vi "Line IR Read.vi"() -> (0 "Line IR Right":bool, 1 "Line IR Left":bool)   [LabVIEW 2013]
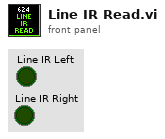
[diagram p1: front panel]
types:
  T1 = typedef "WPI_DigitalInputDevRef.ctl" = cluster{"DevStatus":errorcluster, "DIO Channel":T2, "Digital Module":T3}
  T2 = typedef "FPGA_DIOChannel.ctl" = enum8{"DIO 1", "DIO 2", "DIO 3", "DIO 4", "DIO 5", "DIO 6", "DIO 7", "DIO 8", "DIO 9", "DIO 10", "DIO 11", "DIO 12", "DIO 13", "DIO 14", "Invalid"}
  T3 = typedef "FPGA_TypedefDigitalModule.ctl" = enum16{"Digital Module 1", "Digital Module 2"}
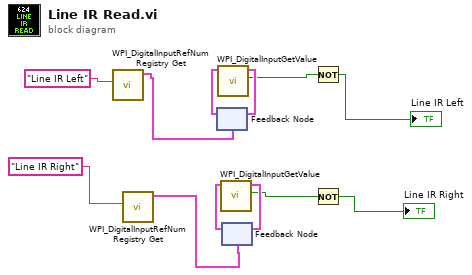
[diagram p0: block diagram]
diagram:
  n1 = call <vilib>:"WPI_DigitalInputRefNum Registry Get.vi"("refnum name"="Line IR Left") -> ("DigitalInputDevRef"=w6:T1)  [unwired: 9 in, 1 out]
  n2 = call <vilib>:"WPI_DigitalInputRefNum Registry Get.vi"("refnum name"="Line IR Right") -> ("DigitalInputDevRef"=w9:T1)  [unwired: 9 in, 1 out]
  n3 = feedback #1(w6) -> (w8:T1)
  n4 = call <vilib>:"WPI_DigitalInputGetValue.vi"("DigitalInputDevRef"=w8) -> ("Value"=w3:bool, "DigitalInputDevRef"=w7:T1)  [unwired: 8 in, 1 out]
  n5 = feedback-in #1(w7) -> ()
  n6 = feedback #2(w9) -> (w11:T1)
  n7 = call <vilib>:"WPI_DigitalInputGetValue.vi"("DigitalInputDevRef"=w11) -> ("Value"=w1:bool, "DigitalInputDevRef"=w10:T1)  [unwired: 8 in, 1 out]
  n8 = feedback-in #2(w10) -> ()
  n9 = Not(x=w3) -> (.not. x?=→"Line IR Left":bool)
  n10 = Not(x=w1) -> (.not. x?=→"Line IR Right":bool)
